vi "MSScript_Act_EncolourCorrectly.vi"(8 "error in (no error)":errorcluster, 11 "MSScript in":refnum<class "MSScript.lvclass">) -> (0 "error out":errorcluster, 3 "MSScript out":refnum<class "MSScript.lvclass">)   [LabVIEW 2018, in "MSScript.lvclass"]
uses:
  MSScript.lvclass
  MSScript.lvclass/MSScript.ctl
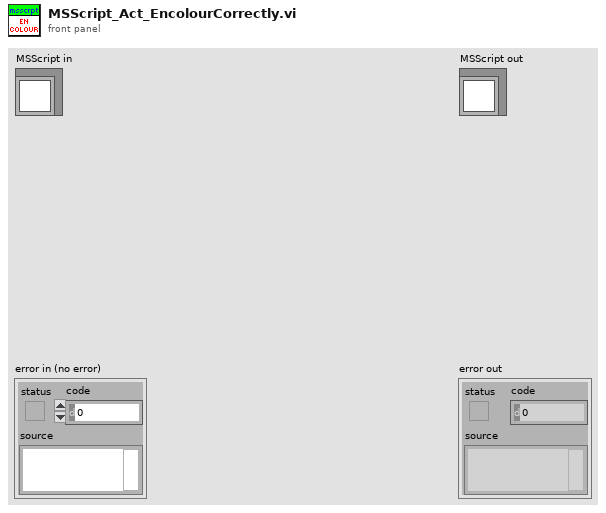
[diagram p1: front panel]
types:
  T1 = cluster{"Colour":u32, "Italic":bool, "Bold":bool}
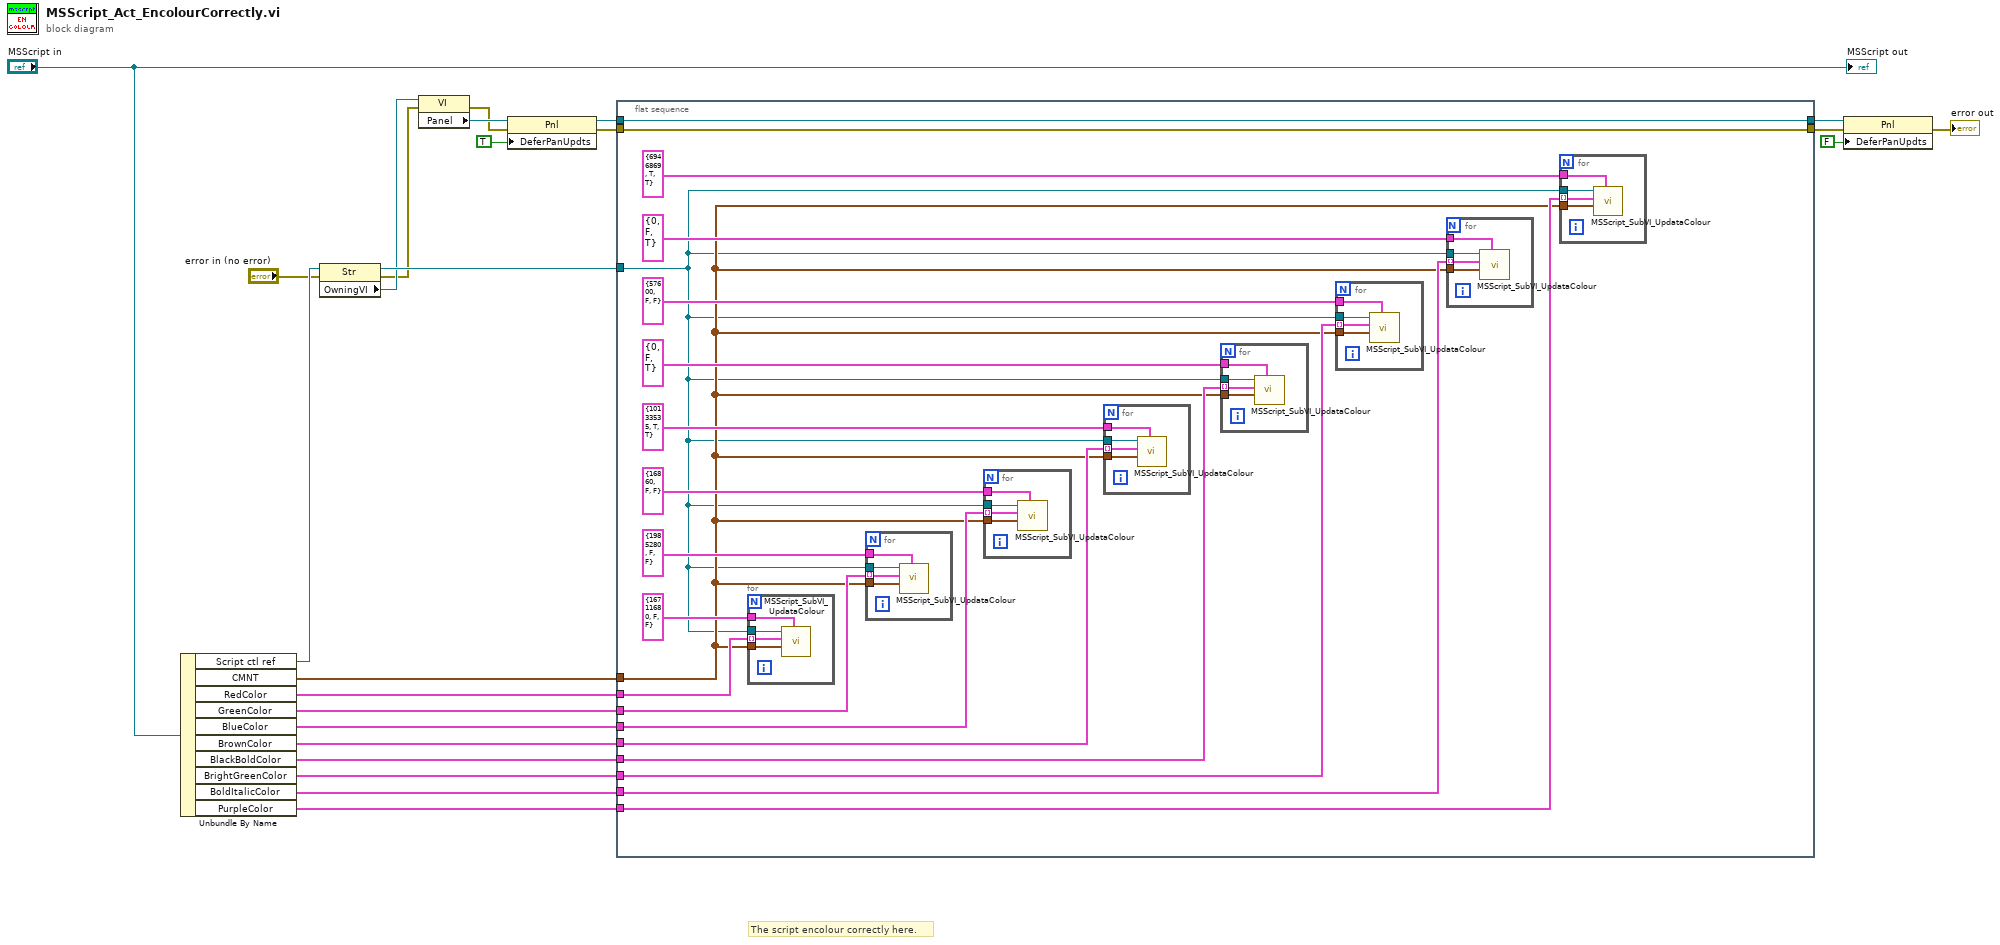
[diagram p0: block diagram]
diagram:
  # "The script encolour correctly here."
  n1 = Unbundle By Name("MSScript in") -> ("Script ctl ref"=w17:refnum<vi>, "CMNT"=w16:cluster{"Start":u32, "End":u32}[], "RedColor"=w23:cluster{"STR":string, "Start":i32}[], "GreenColor"=w22:cluster{"STR":string, "Start":i32}[], "BlueColor"=w21:cluster{"STR":string, "Start":i32}[], "BrownColor"=w20:cluster{"STR":string, "Start":i32}[], "BlackBoldColor"=w19:cluster{"STR":string, "Start":i32}[], "BrightGreenColor"=w18:cluster{"STR":string, "Start":i32}[], "BoldItalicColor"=w15:cluster{"STR":string, "Start":i32}[], "PurpleColor"=w5:cluster{"STR":string, "Start":i32}[])
  n2 = property class="Str"(reference=w17, error in="error in (no error)") -> (reference out=w14:refnum<vi>, error out=w3:errorcluster, "OwningVI"=w13:refnum<vi>)
  n3 = property class="VI"(reference=w13, error in=w3) -> (error out=w2:errorcluster, "Panel"=w12:refnum<vi>)  [unwired: 1 out]
  n4 = property class="Pnl"(reference=w12, error in=w2, "DeferPanUpdts"=TRUE ("Defer Panel Updates")) -> (reference out=w9:refnum<vi>, error out=w10:errorcluster)
  n5 = flat-sequence {
    tunnel: w23 -> [w44]
    tunnel: w22 -> [w43]
    tunnel: w21 -> [w42]
    tunnel: w20 -> [w41]
    tunnel: w19 -> [w40]
    tunnel: w18 -> [w39]
    tunnel: w16 -> [w27]
    tunnel: w15 -> [w31]
    tunnel: w14 -> [w26]
    tunnel: w10 -> [w30]
    tunnel: [w30] -> w7
    tunnel: [w29] -> w8
    tunnel: w9 -> [w29]
    tunnel: w5 -> [w28]
    frame #0 {
      n6 = for {
        tunnel: w26 -> [w76]
        tunnel: w27 -> [w75]
        tunnel: w44 -> [w74] mode=indexing
        tunnel: T1 {"Colour"=16711680, "Italic"=FALSE, "Bold"=FALSE} ("TextProperties") -> [w73]
        n7 = call "MSScript_SubVI_UpdataColour.vi"("TextProperties"=w73, "CMNT in"=w75, "Expression.Section"=w74, "String ref in"=w76) -> ()  [unwired: 8 in]
      }
      n8 = for {
        tunnel: w26 -> [w72]
        tunnel: w27 -> [w71]
        tunnel: w43 -> [w70] mode=indexing
        tunnel: T1 {"Colour"=1985280, "Italic"=FALSE, "Bold"=FALSE} ("TextProperties") -> [w69]
        n9 = call "MSScript_SubVI_UpdataColour.vi"("TextProperties"=w69, "CMNT in"=w71, "Expression.Section"=w70, "String ref in"=w72) -> ()  [unwired: 8 in]
      }
      n10 = for {
        tunnel: w26 -> [w68]
        tunnel: w27 -> [w67]
        tunnel: w42 -> [w66] mode=indexing
        tunnel: T1 {"Colour"=16860, "Italic"=FALSE, "Bold"=FALSE} ("TextProperties") -> [w65]
        n11 = call "MSScript_SubVI_UpdataColour.vi"("TextProperties"=w65, "CMNT in"=w67, "Expression.Section"=w66, "String ref in"=w68) -> ()  [unwired: 8 in]
      }
      n12 = for {
        tunnel: w26 -> [w64]
        tunnel: w27 -> [w63]
        tunnel: w41 -> [w62] mode=indexing
        tunnel: T1 {"Colour"=10133535, "Italic"=TRUE, "Bold"=TRUE} ("TextProperties") -> [w61]
        n13 = call "MSScript_SubVI_UpdataColour.vi"("TextProperties"=w61, "CMNT in"=w63, "Expression.Section"=w62, "String ref in"=w64) -> ()  [unwired: 8 in]
      }
      n14 = for {
        tunnel: w26 -> [w60]
        tunnel: w27 -> [w59]
        tunnel: w40 -> [w58] mode=indexing
        tunnel: T1 {"Colour"=0, "Italic"=FALSE, "Bold"=TRUE} ("TextProperties") -> [w57]
        n15 = call "MSScript_SubVI_UpdataColour.vi"("TextProperties"=w57, "CMNT in"=w59, "Expression.Section"=w58, "String ref in"=w60) -> ()  [unwired: 8 in]
      }
      n16 = for {
        tunnel: w26 -> [w56]
        tunnel: w27 -> [w55]
        tunnel: w39 -> [w54] mode=indexing
        tunnel: T1 {"Colour"=57600, "Italic"=FALSE, "Bold"=FALSE} ("TextProperties") -> [w53]
        n17 = call "MSScript_SubVI_UpdataColour.vi"("TextProperties"=w53, "CMNT in"=w55, "Expression.Section"=w54, "String ref in"=w56) -> ()  [unwired: 8 in]
      }
      n18 = for {
        tunnel: w26 -> [w52]
        tunnel: w27 -> [w51]
        tunnel: w31 -> [w50] mode=indexing
        tunnel: T1 {"Colour"=0, "Italic"=FALSE, "Bold"=TRUE} ("TextProperties") -> [w49]
        n19 = call "MSScript_SubVI_UpdataColour.vi"("TextProperties"=w49, "CMNT in"=w51, "Expression.Section"=w50, "String ref in"=w52) -> ()  [unwired: 8 in]
      }
      n20 = for {
        tunnel: w26 -> [w48]
        tunnel: w27 -> [w47]
        tunnel: w28 -> [w46] mode=indexing
        tunnel: T1 {"Colour"=6946869, "Italic"=TRUE, "Bold"=TRUE} ("TextProperties") -> [w45]
        n21 = call "MSScript_SubVI_UpdataColour.vi"("TextProperties"=w45, "CMNT in"=w47, "Expression.Section"=w46, "String ref in"=w48) -> ()  [unwired: 8 in]
      }
    }
  }
  n22 = property class="Pnl"(reference=w8, error in=w7, "DeferPanUpdts"=FALSE ("Defer Panel Updates")) -> (error out=→"error out":errorcluster)  [unwired: 1 out]
  "MSScript out" <- "MSScript in"
